vi "GetisciFilemeasures_settings_INPUT.vi"(0 "Numero Misure":dbl, 1 "Array ClusterCaratteristicheMisura IN":T1[](array[typedef]), 6 "Azione":string) -> (7 "Array ClusterCaratteristicheMisura OUT":T1[](array[typedef]))   [LabVIEW 2016]
uses:
  TypeDef/ClusterCaratteristicheMisura_INPUT.ctl
  <vilib>/Utility/file.llb/Read Delimited Spreadsheet (string).vi
panel:
  in  "Cluster Caratteriestiche Misura":T1
  out "Lettura file txt":string[][](array[string])
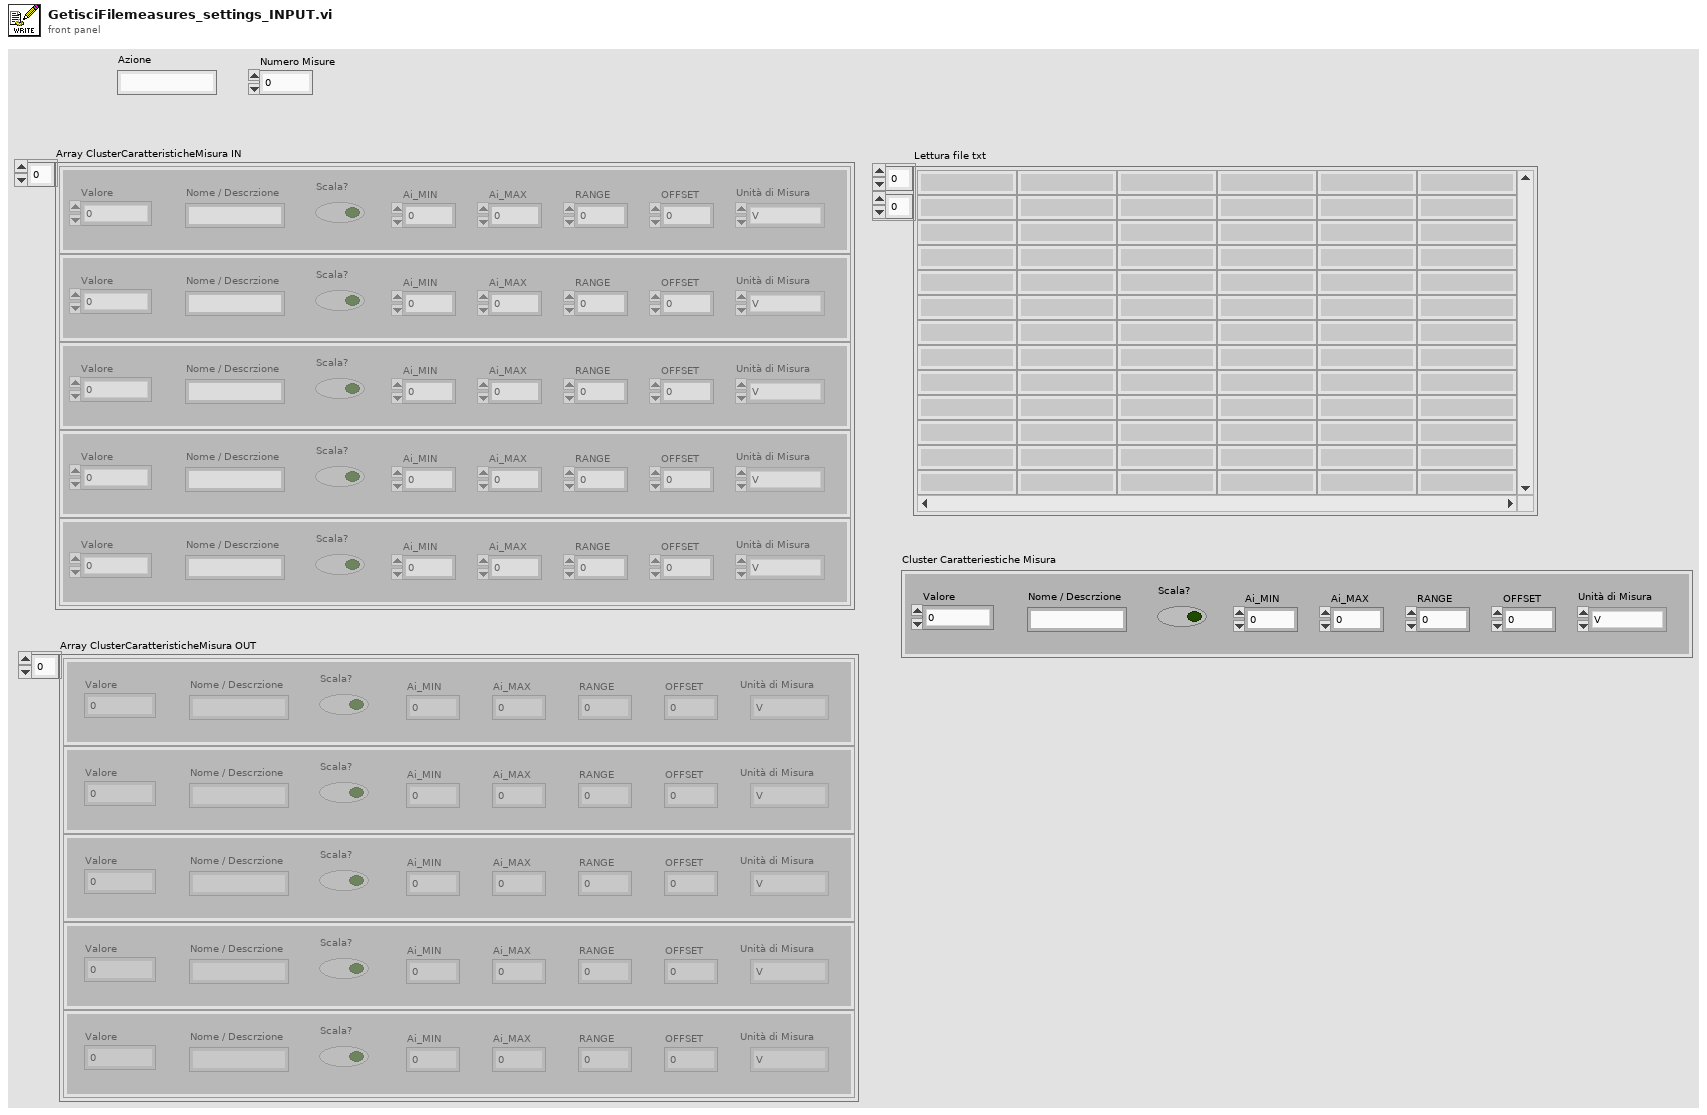
[diagram p1: front panel]
types:
  T1 = typedef "ClusterCaratteristicheMisura_INPUT.ctl" = cluster{"Nome / Descrzione":string, "Scala?":bool, "Ai_MIN":dbl, "Ai_MAX":dbl, "RANGE":dbl, "OFFSET":dbl, "Unità di Misura":T2, "Valore":dbl}
  T2 = typedef "UnitàMisura.ctl" = enum16{"V", "mA", "Bar", "RPM", "m3/s", "m3/min", "m3/h", "l/s", "l/min", "in3/min", "ft3/min", "gpm", "igpm", "igph"}
  T3 = enum16{"open", "replace", "create", "open or create", "replace or create", "replace or create with confirmation"}
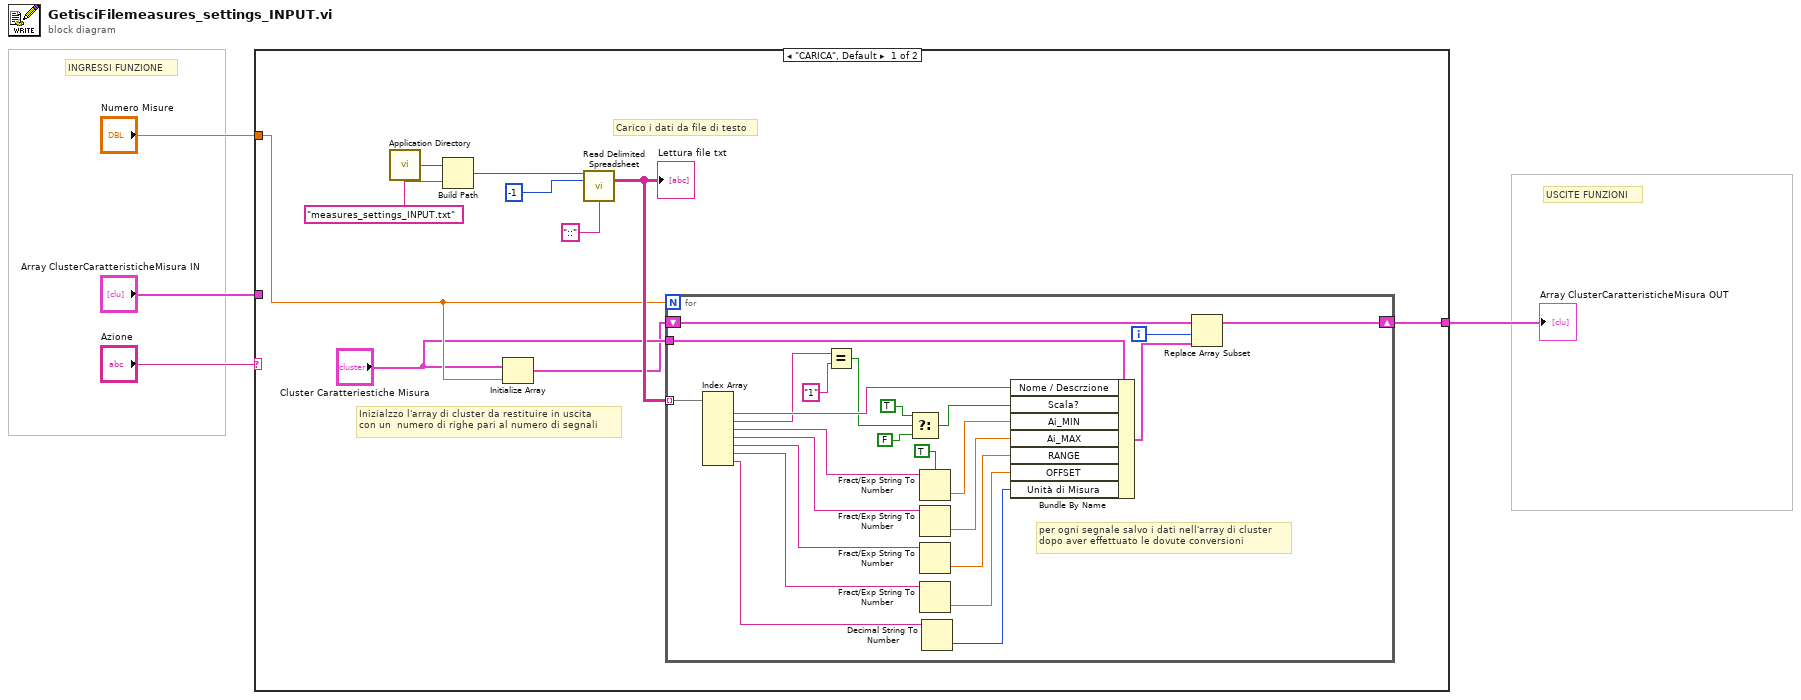
[diagram p0: block diagram]
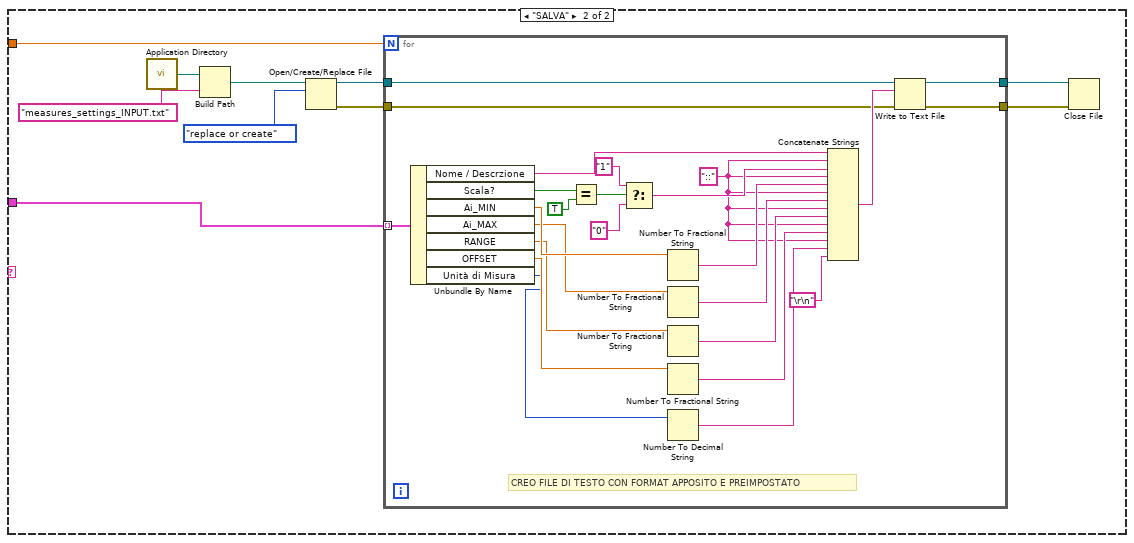
[diagram p2: hidden frame]
diagram:
  # "USCITE FUNZIONI"
  # "INGRESSI FUNZIONE"
  n1 = case shown="\"CARICA\", Default" "Azione" {
    tunnel: "Array ClusterCaratteristicheMisura IN" -> [_ w40]
    tunnel: "Numero Misure" -> [w8 w39]
    tunnel: [w5 _] -> w1
    frame "CARICA", Default {
      # "Inizialzzo l'array di cluster da restituire in uscita\ncon un  numero di righe pari al numero di segnali"
      # "Carico i dati da file di testo"
      n2 = call <vilib>:"Application Directory.vi"() -> ("Application Directory"=w13:path)
      n3 = Build Path(base path=w13, name or relative path="measures_settings_INPUT.txt") -> (appended path=w12:path)
      n4 = Initialize Array("Cluster Caratteriestiche Misura", w8) -> (w6:T1[])
      n5 = call-poly <vilib>:"Read Delimited Spreadsheet.vi"("file path (dialog if empty)"=w12, "number of rows (all:-1)"=-1, "delimiter (\\t)"="::" ("delimiter (\\t)")) -> ("all rows"=w9:string[][])  [unwired: 7 in, 5 out]
      "Lettura file txt" <- w9
      n6 = for {
        N: w8 -> [_]
        tunnel: w9 -> [w38] mode=indexing
        tunnel: "Cluster Caratteriestiche Misura" -> [w19]
        shift-right: [w15] -> w5
        shift-left: w6 -> [w18]
        i -> [w16]
        # "per ogni segnale salvo i dati nell'array di cluster \ndopo aver effettuato le dovute conversioni"
        n7 = Index Array(array=w38) -> (element #1=w37:string, element #2=w36:string, element #3=w29:string, element #4=w27:string, element #5=w26:string, element #6=w25:string, element #7=w21:string)  [unwired: 7 in]
        n8 = Equal?(x=w36, y="1") -> (x = y?=w34:bool)
        n9 = Select(t=TRUE, s=w34, f=FALSE) -> (s? t:f=w31:bool)
        n10 = Fract/Exp String To Number(use system decimal point (T)=TRUE, string=w29) -> (number=w28:dbl)  [unwired: 2 in, 1 out]
        n11 = Fract/Exp String To Number(string=w27) -> (number=w24:dbl)  [unwired: 3 in, 1 out]
        n12 = Fract/Exp String To Number(string=w26) -> (number=w23:dbl)  [unwired: 3 in, 1 out]
        n13 = Fract/Exp String To Number(string=w25) -> (number=w22:dbl)  [unwired: 3 in, 1 out]
        n14 = Decimal String To Number(string=w21) -> (number=w20:i32)  [unwired: 2 in, 1 out]
        n15 = Bundle By Name(cluster=w19, "Nome / Descrzione"=w37, "Scala?"=w31, "Ai_MIN"=w28, "Ai_MAX"=w24, "RANGE"=w23, "OFFSET"=w22, "Unità di Misura"=w20) -> (w17:T1)
        n16 = Replace Array Subset(array=w18, new element=w17, index=w16) -> (w15:T1[])
      }
    }
    frame "SALVA" {
      n17 = call <vilib>:"Application Directory.vi"() -> ("Application Directory"=w48:path)
      n18 = Build Path(base path=w48, name or relative path="measures_settings_INPUT.txt") -> (appended path=w45:path)
      n19 = Open/Create/Replace File(file path (use dialog)=w45, operation (0:open)=T3."replace or create") -> (refnum out=w46:refnum<file>, error out=w42:errorcluster)  [unwired: 4 in, 1 out]
      n20 = for {
        N: w39 -> [_]
        tunnel: w46 -> [w72]
        tunnel: w40 -> [w73] mode=indexing
        tunnel: [w59] -> w43
        tunnel: w42 -> [w58]
        tunnel: [w57] -> w41
        w51 = "::" ("string")
        # "CREO FILE DI TESTO CON FORMAT APPOSITO E PREIMPOSTATO"
        n21 = Unbundle By Name(w73) -> ("Nome / Descrzione"=w66:string, "Scala?"=w71:bool, "Ai_MIN"=w65:dbl, "Ai_MAX"=w64:dbl, "RANGE"=w63:dbl, "OFFSET"=w62:dbl, "Unità di Misura"=w61:T2)
        n22 = Equal?(x=w71, y=TRUE) -> (x = y?=w69:bool)
        n23 = Select(t="1", s=w69, f="0") -> (s? t:f=w56:string)
        n24 = Number To Fractional String(number=w65) -> (F-format string=w55:string)  [unwired: 3 in]
        n25 = Number To Fractional String(number=w64) -> (F-format string=w54:string)  [unwired: 3 in]
        n26 = Number To Fractional String(number=w63) -> (F-format string=w53:string)  [unwired: 3 in]
        n27 = Number To Fractional String(number=w62) -> (F-format string=w52:string)  [unwired: 3 in]
        n28 = Number To Decimal String(number=w61) -> (decimal integer string=w50:string)  [unwired: 1 in]
        n29 = Concatenate Strings(w66, w51, w56, w51, w55, w51, w54, w51, w53, w51, w52, w51, w50, "\r\n") -> (w60:string)
        n30 = Write to Text File(file (use dialog)=w72, text=w60, error in=w58) -> (refnum out=w59:refnum<file>, error out=w57:errorcluster)  [unwired: 1 in, 1 out]
      }
      n31 = Close File(refnum=w43, error in=w41) -> ()  [unwired: 2 out]
    }
  }
  "Array ClusterCaratteristicheMisura OUT" <- w1
